vi "Start Log_PID.vi"(8 "Error In":errorcluster, 11 "Log Prefix":string) -> (0 "Error Out":errorcluster, 3 "refnum out":refnum<file>)   [LabVIEW 2015]
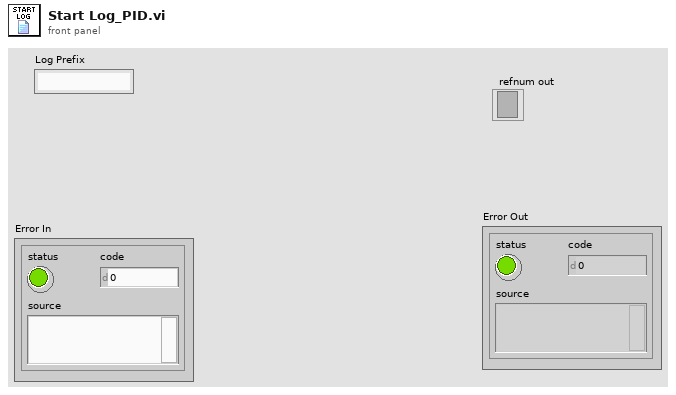
[diagram p1: front panel]
types:
  T1 = enum16{"open", "replace", "create", "open or create", "replace or create", "replace or create with confirmation"}
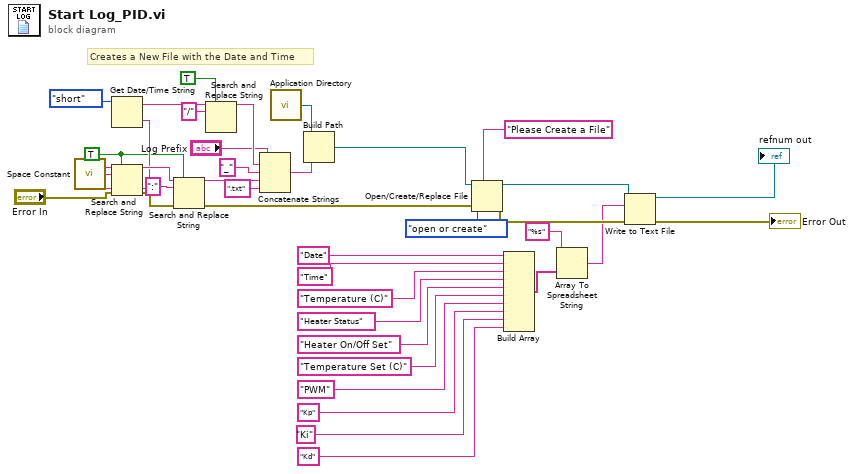
[diagram p0: block diagram]
diagram:
  w27 = TRUE
  # "Creates a New File with the Date and Time"
  n1 = call <vilib>:"Space Constant.vi"() -> ("String"=w30:string)
  n2 = Get Date/Time String(date format (0)=enum16{"short", "long", "abbreviated"}."short") -> (date string=w37:string, time string=w29:string)  [unwired: 2 in]
  n3 = Search and Replace String(replace all?=w27, input string=w29, search string=w30, error in="Error In") -> (result string=w35:string, error out=w13:errorcluster)  [unwired: 4 in, 2 out]
  n4 = Search and Replace String(replace all?=w27, input string=w35, search string=":", error in=w13) -> (result string=w28:string, error out=w12:errorcluster)  [unwired: 4 in, 2 out]
  n5 = Search and Replace String(replace all?=TRUE ("replace all? (F)"), input string=w37, search string="/") -> (result string=w31:string)  [unwired: 5 in, 3 out]
  n6 = Concatenate Strings("Log Prefix", w31, "_" ("string"), w28, ".txt" ("string")) -> (w39:string)
  n7 = call <vilib>:"Application Directory.vi"() -> ("Application Directory"=w25:path)
  n8 = Build Path(base path=w25, name or relative path=w39) -> (appended path=w16:path)
  n9 = Open/Create/Replace File(file path (use dialog)=w16, error in=w12, prompt="Please Create a File", operation (0:open)=T1."open or create") -> (refnum out=w23:refnum<file>, error out=w22:errorcluster)  [unwired: 2 in, 1 out]
  n10 = Build Array("Date", "Time", "Temperature (C)", "Heater Status", "Heater On/Off Set", "Temperature Set (C)", "PWM", "Kp", "Ki", "Kd") -> (w20:string[])
  n11 = Array To Spreadsheet String(array=w20, 3:"%s" ("format string")) -> (spreadsheet string=w19:string)  [unwired: 1 in]
  n12 = Write to Text File(file (use dialog)=w23, text=w19, error in=w22) -> (refnum out=→"refnum out":refnum<file>, error out=→"Error Out":errorcluster)  [unwired: 1 in, 1 out]
